vi "Write VI Ref.vi"(8 "error in (no error)":errorcluster, 10 "VI Ref":refnum<vi>, 11 "Chat Window Controller in":refnum<class "Chat Window Controller.lvclass">) -> (0 "error out":errorcluster, 3 "Chat Window Controller out":refnum<class "Chat Window Controller.lvclass">)   [LabVIEW 2020, in "Chat Window UI Controller.lvlib" / "Chat Window Controller.lvclass"]
uses:
  Chat Window Controller.lvclass
  Chat Window Controller.lvclass/Chat Window Controller.ctl
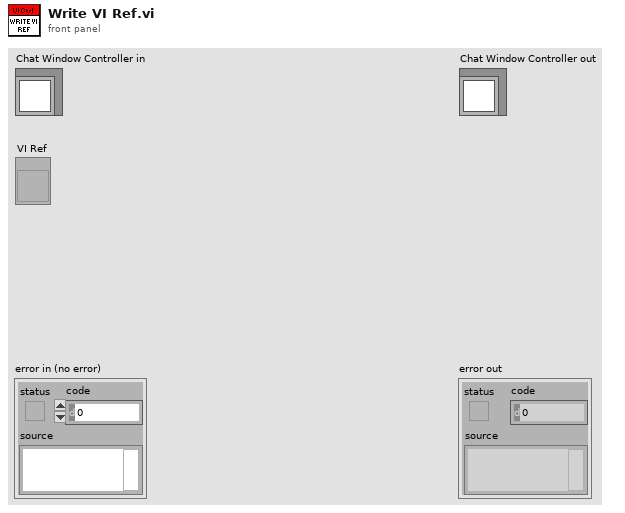
[diagram p1: front panel]
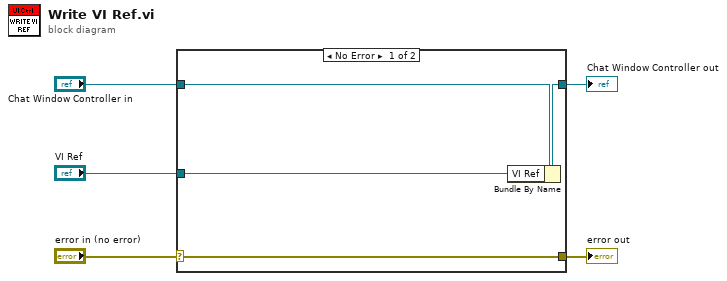
[diagram p0: block diagram]
diagram:
  n1 = case shown="No Error" "error in (no error)" {
    selector: "error in (no error)" -> [w9 w10]
    tunnel: [w9 w10] -> w4
    tunnel: [w7 w11] -> w2
    tunnel: "Chat Window Controller in" -> [w8 w11]
    tunnel: "VI Ref" -> [w6 _]
    frame No Error {
      n2 = Bundle By Name(cluster=w8, "VI Ref"=w6) -> (w7:refnum<class "Chat Window Controller.lvclass">)
    }
    frame Error {
    }
  }
  "error out" <- w4
  "Chat Window Controller out" <- w2
